vi "HAB Climber.vi"   [LabVIEW 2018]
uses:
  <vilib>/Rock Robotics/SystemInterfaces/DIO/FPGA_DIOChannel.ctl
  <vilib>/Rock Robotics/WPI/ThirdParty/Phoenix-LabVIEW/Motor Controller/Controls/CTRE_Phoenix_MotorControl_ControlMode.ctl
  HAB Climber Global.vi
  <vilib>/Rock Robotics/WPI/Switch/WPI_SwitchOpenLimit.vi
  Times/Times Global.vi
  Controllers/Driver Controller/Driver Controller Global.vi
  Cargo Intake/Cargo Intake Global.vi
types:
  T1 = typedef "FPGA_DIOChannel.ctl" = enum8{"DIO 0", "DIO 1", "DIO 2", "DIO 3", "DIO 4", "DIO 5", "DIO 6", "DIO 7", "DIO 8", "DIO 9", "DIO MXP 0", "DIO MXP 1", "DIO MXP 2", "DIO MXP 3", "DIO MXP 4", "DIO MXP 5", "DIO MXP 6", "DIO MXP 7", "DIO MXP 8", "DIO MXP 9", "DIO MXP 10", "DIO MXP 11", "DIO MXP 12", "DIO MXP 13", "DIO MXP 14", "DIO MXP 15", "SPI Port CS1", "SPI Port CS2", "SPI Port CS3", "SPI Port MISO", "SPI Port MOSI", "Invalid"}
  T2 = enum16{"HAB Climber Full Manual Mode", "HAB Climber Manual Mode", "HAB Climber Automated Mode", "HAB Climber Fully Automated Mode"}
  T3 = typedef "WPI_SwitchDevRef.ctl" = cluster{"DevStatus":errorcluster, "DIO Channel":T1, "CntIndex":T4, "Normally Closed":bool}
  T4 = typedef "FPGA_CounterCtrSystemIndex.ctl" = enum8{"Ctr 0", "Ctr 1", "Ctr 2", "Ctr 3", "Ctr 4", "Ctr 5", "Ctr 6", "Ctr 7", "Invalid"}
  T5 = typedef "WPI_MotorControlDeviceRef.ctl" = cluster{"DeviceStatus":errorcluster, "Type":T6, "PWM":cluster{"PWM Channel":T7, "DeadBand":T8}, "CAN":cluster{"Device Number":u8, "SetOutput VI Ref":variant, "GetOutput VI Ref":variant, "Enable VI Ref":variant, "Disable VI Ref":variant, "Data":variant}, "Invert":bool, "DIO PWM":cluster{"PWM \"Enable\" Channel":T7, "DIOChannel":T1, "PWM Rate":dbl}}
  T6 = typedef "WPI_MotorControlType.ctl" = enum16{"PWM", "CAN", "DIO PWM"}
  T7 = typedef "FPGA_DIOPWMChannel.ctl" = enum8{"PWM 0", "PWM 1", "PWM 2", "PWM 3", "PWM 4", "PWM 5", "PWM 6", "PWM 7", "PWM 8", "PWM 9", "PWM MXP 0", "PWM MXP 1", "PWM MXP 2", "PWM MXP 3", "PWM MXP 4", "PWM MXP 5", "PWM MXP 6", "PWM MXP 7", "PWM MXP 8", "PWM MXP 9", "Invalid"}
  T8 = typedef "WPI_PWMDeadband.ctl" = cluster{"Name":string, "maxPositivePwm":i32, "minPositivePwm":i32, "centerPwm":i32, "maxNegativePwm":i32, "minNegativePwm":i32, "angularRange":u16}
  T9 = typedef "Control 3.ctl" = dbl
  T10 = typedef "CTRE_Phoenix_MotorControl_ControlMode.ctl" = u16
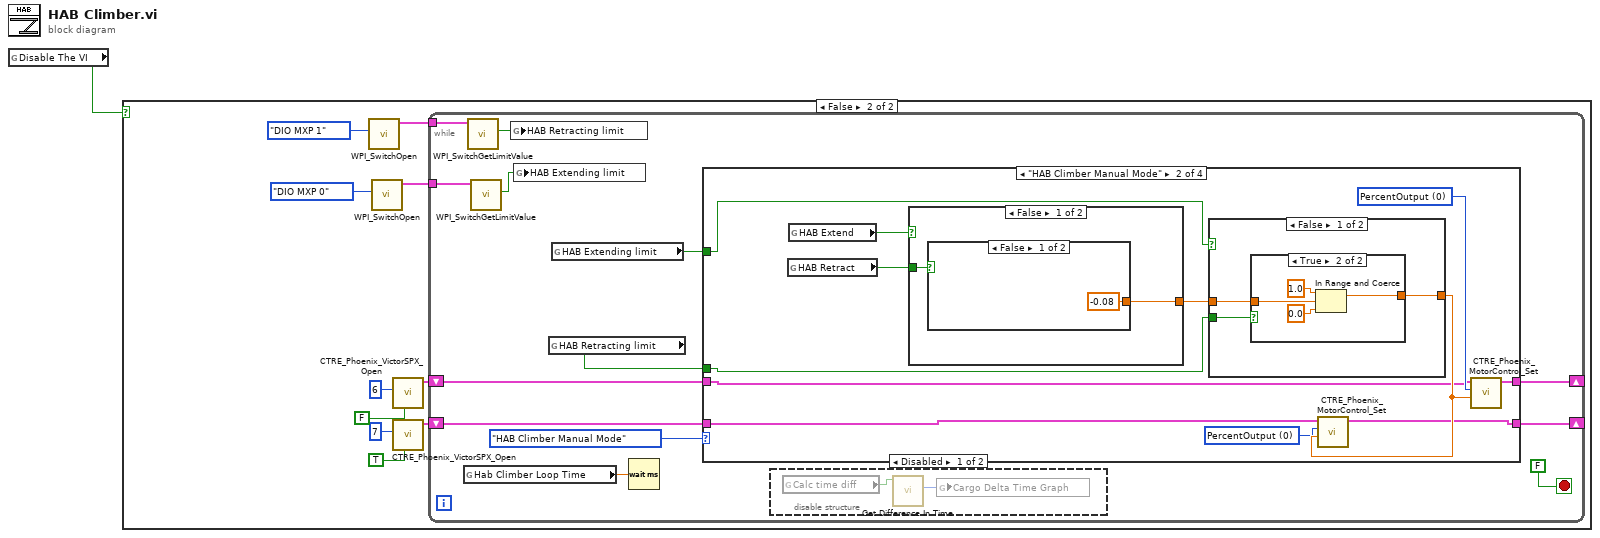
[diagram p0: block diagram]
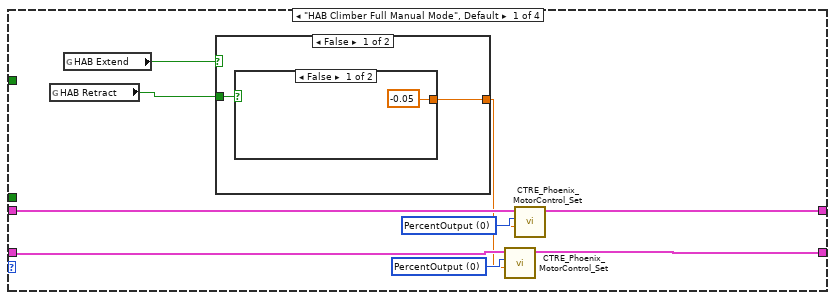
[diagram p4: hidden frame]
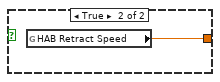
[diagram p5: hidden frame]
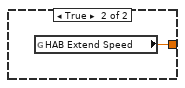
[diagram p6: hidden frame]
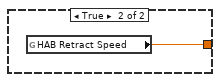
[diagram p7: hidden frame]
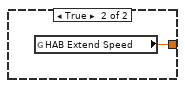
[diagram p8: hidden frame]
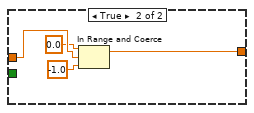
[diagram p10: hidden frame]
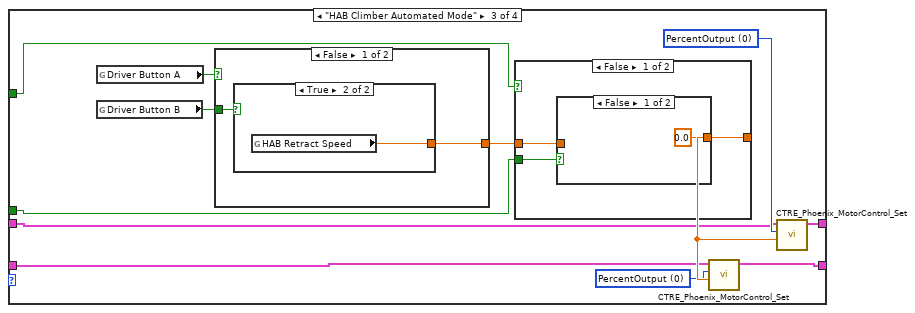
[diagram p11: hidden frame]
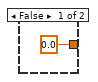
[diagram p12: hidden frame]
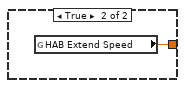
[diagram p13: hidden frame]
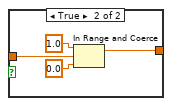
[diagram p14: hidden frame]
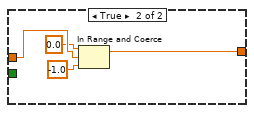
[diagram p15: hidden frame]
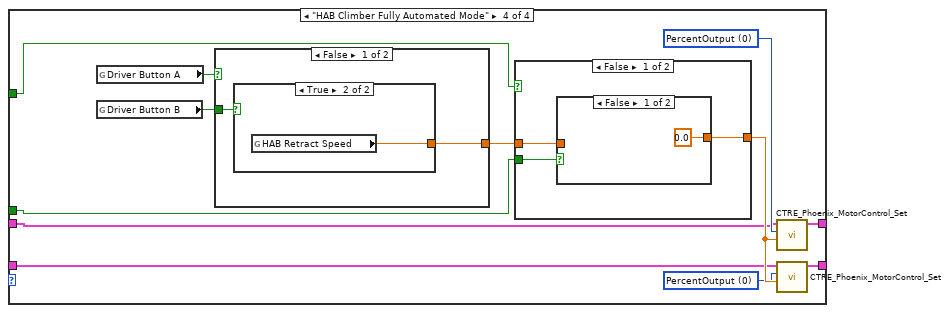
[diagram p16: hidden frame]
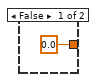
[diagram p17: hidden frame]
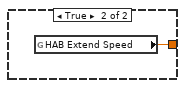
[diagram p18: hidden frame]
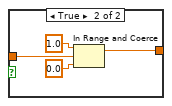
[diagram p19: hidden frame]
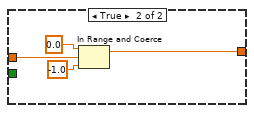
[diagram p20: hidden frame]
diagram:
  n1 = global read "HAB Climber Global.vi" "Disable The VI"() -> (w1:bool)
  n2 = case shown="False" w1 {
    frame True {
    }
    frame False {
      n3 = call-poly <vilib>:"WPI_SwitchOpen.vi"("DIO Channel"=FPGA_DIOChannel."DIO MXP 1") -> ("SwitchDevRef"=w5:T3)  [unwired: 9 in, 1 out]
      n4 = call-poly <vilib>:"WPI_SwitchOpen.vi"("DIO Channel"=FPGA_DIOChannel."DIO MXP 0") -> ("SwitchDevRef"=w4:T3)  [unwired: 9 in, 1 out]
      n5 = call <vilib>:"CTRE_Phoenix_VictorSPX_Open.vi"("Invert"=FALSE, "Device Number"=u8 6) -> ("CAN Talon SRX Ref"=w11:T5)  [unwired: 8 in, 1 out]
      n6 = call <vilib>:"CTRE_Phoenix_VictorSPX_Open.vi"("Invert"=TRUE, "Device Number"=u8 7) -> ("CAN Talon SRX Ref"=w9:T5)  [unwired: 8 in, 1 out]
      n7 = while {
        shift-right: [w19] -> _
        shift-left: w11 -> [w21]
        shift-right: [w18] -> _
        shift-left: w9 -> [w20]
        tunnel: w5 -> [w17]
        tunnel: w4 -> [w16]
        stop <- FALSE stop-if-true
        n8 = global read "Times Global.vi" "Hab Climber Loop Time"() -> (w24:T9)
        n9 = call <vilib>:"WPI_SwitchGetLimitValue.vi"("SwitchDevRef"=w17) -> ("Switch Pressed"=w12:bool)  [unwired: 8 in, 2 out]
        n10 = call <vilib>:"WPI_SwitchGetLimitValue.vi"("SwitchDevRef"=w16) -> ("Switch Pressed"=w13:bool)  [unwired: 8 in, 2 out]
        n11 = global write "HAB Climber Global.vi" "HAB Retracting limit"(w12) -> ()
        n12 = global write "HAB Climber Global.vi" "HAB Extending limit"(w13) -> ()
        n13 = global read "HAB Climber Global.vi" "HAB Retracting limit"() -> (w14:bool)
        n14 = global read "HAB Climber Global.vi" "HAB Extending limit"() -> (w15:bool)
        n15 = Wait (ms)(milliseconds to wait=w24) -> ()  [unwired: 1 out]
        n16 = case shown="\"HAB Climber Manual Mode\"" T2."HAB Climber Manual Mode" ("Mode") {
          tunnel: w21 -> [w32 w48 w75 w104]
          tunnel: w20 -> [w33 w47 w74 w103]
          tunnel: [w30 w46 w73 w102] -> w19
          tunnel: [w29 w45 w72 w101] -> w18
          tunnel: w15 -> [_ w44 w71 w100]
          tunnel: w14 -> [_ w43 w70 w99]
          frame "HAB Climber Full Manual Mode", Default {
            w34 = T10 0 items=["PercentOutput"=0, "Position"=1, "Velocity"=2, "Current"=3, "Follower"=5, "MotionProfile"=6, "MotionMagic"=7, "MotionProfileArc"=10, "Disabled"=15] ("Control Mode")
            w35 = T10 0 items=["PercentOutput"=0, "Position"=1, "Velocity"=2, "Current"=3, "Follower"=5, "MotionProfile"=6, "MotionMagic"=7, "MotionProfileArc"=10, "Disabled"=15] ("Control Mode")
            n17 = global read "HAB Climber Global.vi" "HAB Retract"() -> (w27:bool)
            n18 = global read "HAB Climber Global.vi" "HAB Extend"() -> (w28:bool)
            n19 = case shown="False" w28 {
              tunnel: w27 -> [w37 _]
              tunnel: [w36 w40] -> w31
              frame False {
                n20 = case shown="False" w37 {
                  tunnel: [-0.05 w39] -> w36
                  frame False {
                  }
                  frame True {
                    n21 = global read "HAB Climber Global.vi" "HAB Retract Speed"() -> (w39:dbl)
                  }
                }
              }
              frame True {
                n22 = global read "HAB Climber Global.vi" "HAB Extend Speed"() -> (w40:dbl)
              }
            }
            n23 = call <vilib>:"CTRE_Phoenix_MotorControl_Set.vi"("Output"=w31, "Control Mode"=w34, "PhoenixMotorControlDevRef"=w33) -> ("PhoenixMotorControlDevRef"=w29:T5)  [unwired: 7 in, 1 out]
            n24 = call <vilib>:"CTRE_Phoenix_MotorControl_Set.vi"("Output"=w31, "Control Mode"=w35, "PhoenixMotorControlDevRef"=w32) -> ("PhoenixMotorControlDevRef"=w30:T5)  [unwired: 7 in, 1 out]
          }
          frame "HAB Climber Manual Mode" {
            w49 = T10 0 items=["PercentOutput"=0, "Position"=1, "Velocity"=2, "Current"=3, "Follower"=5, "MotionProfile"=6, "MotionMagic"=7, "MotionProfileArc"=10, "Disabled"=15] ("Control Mode")
            w51 = T10 0 items=["PercentOutput"=0, "Position"=1, "Velocity"=2, "Current"=3, "Follower"=5, "MotionProfile"=6, "MotionMagic"=7, "MotionProfileArc"=10, "Disabled"=15] ("Control Mode")
            n25 = global read "HAB Climber Global.vi" "HAB Retract"() -> (w41:bool)
            n26 = global read "HAB Climber Global.vi" "HAB Extend"() -> (w42:bool)
            n27 = case shown="False" w42 {
              tunnel: w41 -> [w54 _]
              tunnel: [w53 w57] -> w52
              frame False {
                n28 = case shown="False" w54 {
                  tunnel: [-0.08 w56] -> w53
                  frame False {
                  }
                  frame True {
                    n29 = global read "HAB Climber Global.vi" "HAB Retract Speed"() -> (w56:dbl)
                  }
                }
              }
              frame True {
                n30 = global read "HAB Climber Global.vi" "HAB Extend Speed"() -> (w57:dbl)
              }
            }
            n31 = case shown="False" w44 {
              tunnel: w52 -> [w59 w69]
              tunnel: [w60 w66] -> w50
              tunnel: w43 -> [w58 _]
              frame False {
                n32 = case shown="True" w58 {
                  tunnel: [w61 w65] -> w60
                  tunnel: w59 -> [w61 w64]
                  frame False {
                  }
                  frame True {
                    n33 = In Range and Coerce(upper limit=1.0, x=w64, lower limit=0.0) -> (coerced(x)=w65:dbl)  [unwired: 1 out]
                  }
                }
              }
              frame True {
                n34 = In Range and Coerce(upper limit=0.0, x=w69, lower limit=-1.0) -> (coerced(x)=w66:dbl)  [unwired: 1 out]
              }
            }
            n35 = call <vilib>:"CTRE_Phoenix_MotorControl_Set.vi"("Output"=w50, "Control Mode"=w49, "PhoenixMotorControlDevRef"=w47) -> ("PhoenixMotorControlDevRef"=w45:T5)  [unwired: 7 in, 1 out]
            n36 = call <vilib>:"CTRE_Phoenix_MotorControl_Set.vi"("Output"=w50, "Control Mode"=w51, "PhoenixMotorControlDevRef"=w48) -> ("PhoenixMotorControlDevRef"=w46:T5)  [unwired: 7 in, 1 out]
          }
          frame "HAB Climber Automated Mode" {
            w76 = T10 0 items=["PercentOutput"=0, "Position"=1, "Velocity"=2, "Current"=3, "Follower"=5, "MotionProfile"=6, "MotionMagic"=7, "MotionProfileArc"=10, "Disabled"=15] ("Control Mode")
            w77 = T10 0 items=["PercentOutput"=0, "Position"=1, "Velocity"=2, "Current"=3, "Follower"=5, "MotionProfile"=6, "MotionMagic"=7, "MotionProfileArc"=10, "Disabled"=15] ("Control Mode")
            n37 = global read "Driver Controller Global.vi" "Driver Button A"() -> (w79:bool)
            n38 = global read "Driver Controller Global.vi" "Driver Button B"() -> (w78:bool)
            n39 = case shown="False" w79 {
              tunnel: w78 -> [w83 _]
              tunnel: [w82 w86] -> w80
              frame False {
                n40 = case shown="True" w83 {
                  tunnel: [0.0 w85] -> w82
                  frame False {
                  }
                  frame True {
                    n41 = global read "HAB Climber Global.vi" "HAB Retract Speed"() -> (w85:dbl)
                  }
                }
              }
              frame True {
                n42 = global read "HAB Climber Global.vi" "HAB Extend Speed"() -> (w86:dbl)
              }
            }
            n43 = case shown="False" w71 {
              tunnel: w80 -> [w88 w98]
              tunnel: [w89 w95] -> w81
              tunnel: w70 -> [w87 _]
              frame False {
                n44 = case shown="False" w87 {
                  tunnel: [0.0 w94] -> w89
                  tunnel: w88 -> [_ w93]
                  frame False {
                  }
                  frame True {
                    n45 = In Range and Coerce(upper limit=1.0, x=w93, lower limit=0.0) -> (coerced(x)=w94:dbl)  [unwired: 1 out]
                  }
                }
              }
              frame True {
                n46 = In Range and Coerce(upper limit=0.0, x=w98, lower limit=-1.0) -> (coerced(x)=w95:dbl)  [unwired: 1 out]
              }
            }
            n47 = call <vilib>:"CTRE_Phoenix_MotorControl_Set.vi"("Output"=w81, "Control Mode"=w76, "PhoenixMotorControlDevRef"=w74) -> ("PhoenixMotorControlDevRef"=w72:T5)  [unwired: 7 in, 1 out]
            n48 = call <vilib>:"CTRE_Phoenix_MotorControl_Set.vi"("Output"=w81, "Control Mode"=w77, "PhoenixMotorControlDevRef"=w75) -> ("PhoenixMotorControlDevRef"=w73:T5)  [unwired: 7 in, 1 out]
          }
          frame "HAB Climber Fully Automated Mode" {
            w105 = T10 0 items=["PercentOutput"=0, "Position"=1, "Velocity"=2, "Current"=3, "Follower"=5, "MotionProfile"=6, "MotionMagic"=7, "MotionProfileArc"=10, "Disabled"=15] ("Control Mode")
            w106 = T10 0 items=["PercentOutput"=0, "Position"=1, "Velocity"=2, "Current"=3, "Follower"=5, "MotionProfile"=6, "MotionMagic"=7, "MotionProfileArc"=10, "Disabled"=15] ("Control Mode")
            n49 = global read "Driver Controller Global.vi" "Driver Button A"() -> (w108:bool)
            n50 = global read "Driver Controller Global.vi" "Driver Button B"() -> (w107:bool)
            n51 = case shown="False" w108 {
              tunnel: w107 -> [w112 _]
              tunnel: [w111 w115] -> w109
              frame False {
                n52 = case shown="True" w112 {
                  tunnel: [0.0 w114] -> w111
                  frame False {
                  }
                  frame True {
                    n53 = global read "HAB Climber Global.vi" "HAB Retract Speed"() -> (w114:dbl)
                  }
                }
              }
              frame True {
                n54 = global read "HAB Climber Global.vi" "HAB Extend Speed"() -> (w115:dbl)
              }
            }
            n55 = case shown="False" w100 {
              tunnel: w109 -> [w117 w127]
              tunnel: [w118 w124] -> w110
              tunnel: w99 -> [w116 _]
              frame False {
                n56 = case shown="False" w116 {
                  tunnel: [0.0 w123] -> w118
                  tunnel: w117 -> [_ w122]
                  frame False {
                  }
                  frame True {
                    n57 = In Range and Coerce(upper limit=1.0, x=w122, lower limit=0.0) -> (coerced(x)=w123:dbl)  [unwired: 1 out]
                  }
                }
              }
              frame True {
                n58 = In Range and Coerce(upper limit=0.0, x=w127, lower limit=-1.0) -> (coerced(x)=w124:dbl)  [unwired: 1 out]
              }
            }
            n59 = call <vilib>:"CTRE_Phoenix_MotorControl_Set.vi"("Output"=w110, "Control Mode"=w106, "PhoenixMotorControlDevRef"=w104) -> ("PhoenixMotorControlDevRef"=w102:T5)  [unwired: 7 in, 1 out]
            n60 = call <vilib>:"CTRE_Phoenix_MotorControl_Set.vi"("Output"=w110, "Control Mode"=w105, "PhoenixMotorControlDevRef"=w103) -> ("PhoenixMotorControlDevRef"=w101:T5)  [unwired: 7 in, 1 out]
          }
        }
        n61 = disable-structure shown="Disabled" {
          frame Disabled {
            n62 = global read "Cargo Intake Global.vi" "Calc time diff"() -> (w26:bool)
            n63 = call "Get Difference In Time.vi"("Calculate Time Difference"=w26) -> ("Delta Time over Time"=w25:u32)  [unwired: 9 in, 1 out]
            n64 = global write "Times Global.vi" "Cargo Delta Time Graph"(w25) -> ()
          }
          frame Enabled {
          }
        }
      }
    }
  }
